vi "Archive Headers DAO.vi"(7 "Archive File Type":T1, 8 "error in (no error)":errorcluster, 9 "Headers In":string[](array[string]), 10 "LogFile Type":T2=enum."DLL  Errors", 11 "Actions":T3) -> (0 "error out":errorcluster, 2 "Record Out":string)   [LabVIEW 2013]
uses:
  Data Access Objects/Metadata/DAO Actions.ctl
  LogFileType.ctl
  Archive File Type.ctl
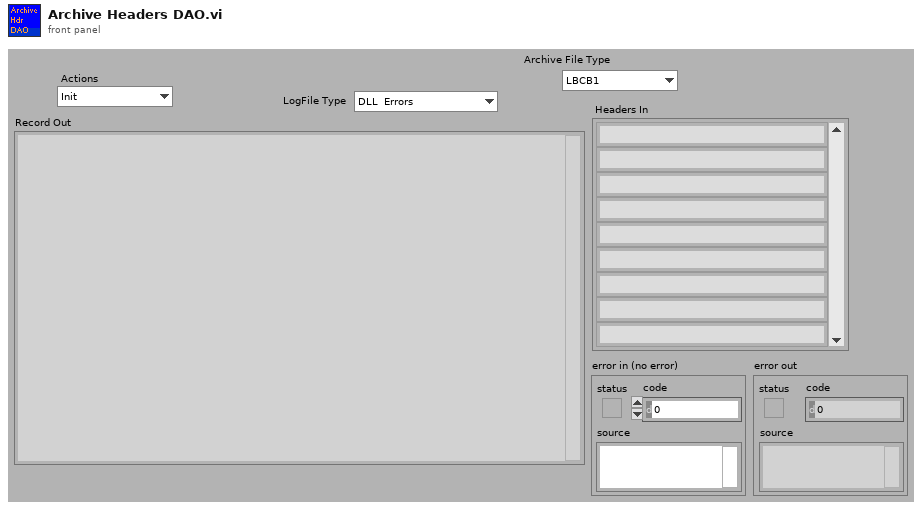
[diagram p1: front panel]
types:
  T1 = typedef "Archive File Type.ctl" = enum16{"LBCB1", "LBCB2", "ExternalSensors", "Combined"}
  T2 = typedef "LogFileType.ctl" = enum16{"Continuous", "Step", "Volts", "Offsets", "DLL  Errors", "Snapshot", "Commands", "StiffnessUpdates", "Debug", "End List"}
  T3 = typedef "DAO Actions.ctl" = enum16{"Init", "Get", "Set"}
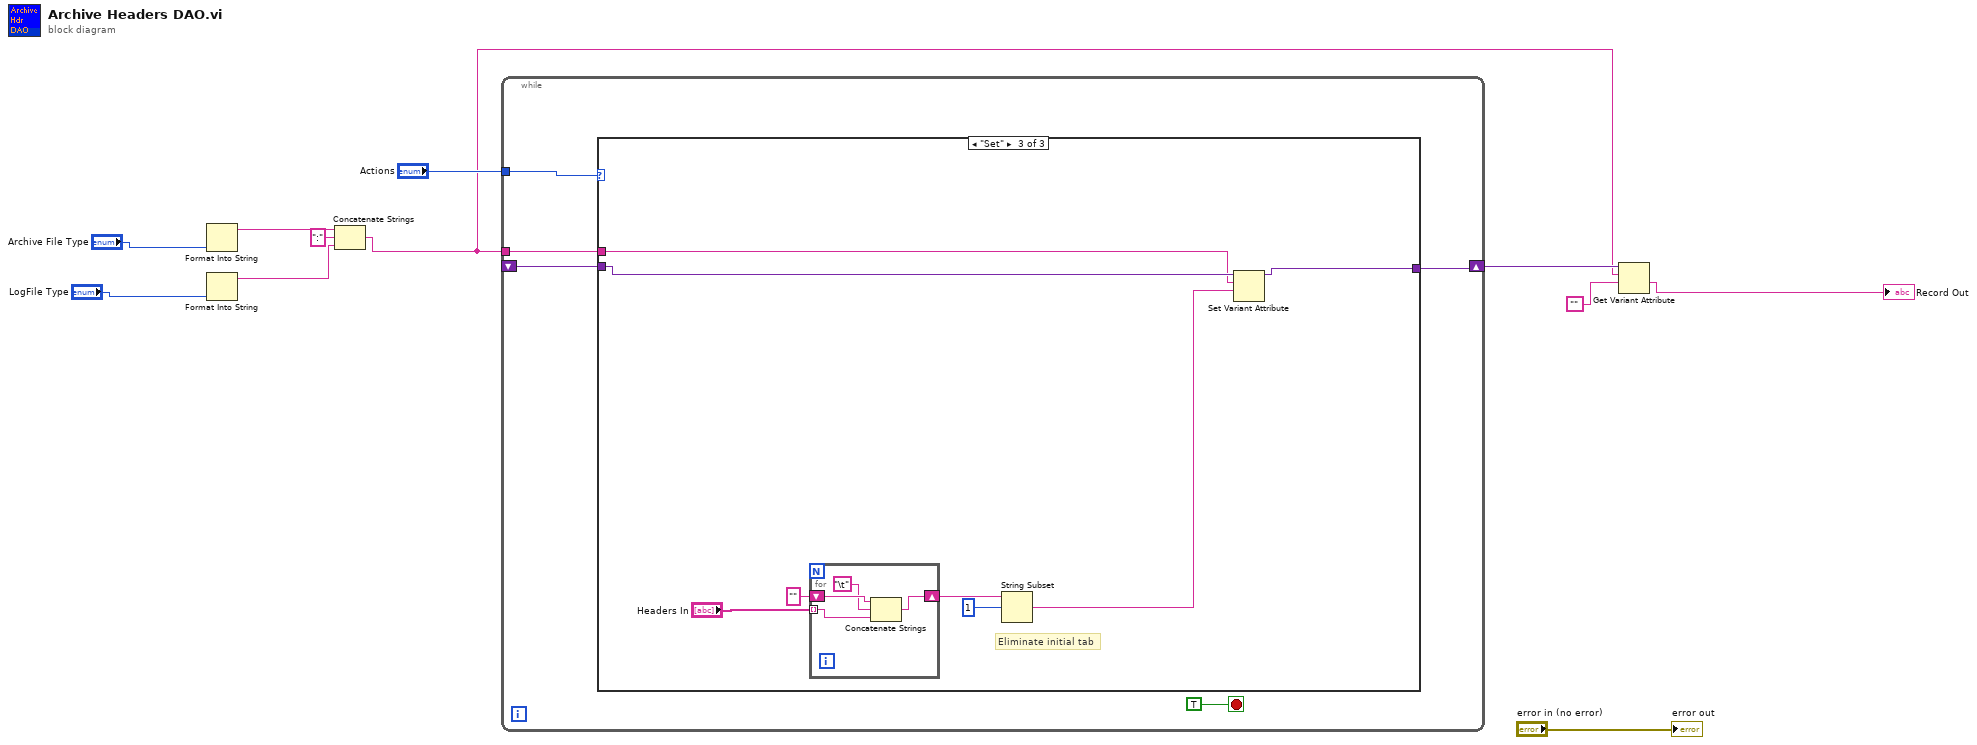
[diagram p0: block diagram]
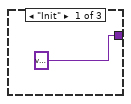
[diagram p2: hidden frame]
diagram:
  n1 = Format Into String("Archive File Type") -> (resulting string=w4:string)  [unwired: 3 in, 1 out]
  n2 = Format Into String("LogFile Type") -> (resulting string=w6:string)  [unwired: 3 in, 1 out]
  n3 = Concatenate Strings(w4, ":" ("string"), w6) -> (w1:string)
  n4 = while {
    tunnel: "Actions" -> [w15]
    shift-right: [w13] -> w9
    shift-left: _ -> [w14]
    tunnel: w1 -> [w12]
    stop <- TRUE stop-if-true
    n5 = case shown="\"Set\"" w15 {
      tunnel: w14 -> [_ w18 w20]
      tunnel: [variant w18 w21] -> w13
      tunnel: w12 -> [_ _ w19]
      frame "Init" {
      }
      frame "Get" {
      }
      frame "Set" {
        # "Eliminate initial tab"
        n6 = for {
          tunnel: "Headers In" -> [w27] mode=indexing
          shift-right: [w30] -> w25
          shift-left: "" -> [w29]
          n7 = Concatenate Strings(w29, "\t", w27) -> (w30:string)
        }
        n8 = String Subset(string=w25, offset (0)=1) -> (substring=w22:string)  [unwired: 1 out]
        n9 = Set Variant Attribute(Variant=w20, name=w19, value=w22) -> (Variant out=w21:variant)  [unwired: 1 in, 2 out]
      }
    }
  }
  n10 = Get Variant Attribute(Variant=w9, name=w1, default value (empty Variant)="") -> (value=→"Record Out":string)  [unwired: 1 in, 3 out]
  "error out" <- "error in (no error)"
